vi "Test Convert.vi"(11 "Error in":errorcluster) -> (15 "Error out":errorcluster)   [LabVIEW 2020, in "CelsiusToFarenheitTests.lvlib"]
doc: "This VI is to validate Celsius to farenheit"
uses:
  CelsiusToFarenheitTests.lvlib
  <vilib>/SLL Drona/APIs/Stimulus/ControlValue/ValueSignalByPathString.vi
  <vilib>/SLL Drona/APIs/Assert/AssertControlValue/AlmostEqual.vi
  <vilib>/SLL Drona/APIs/Stimulus/VI/CloseVI.vi
  <vilib>/SLL Drona/Drona.lvlib
  <vilib>/addons/_JKI Toolkits/Caraya/classes/Test/Test.lvclass
  <vilib>/SLL Drona/APIs/Stimulus/ControlValue/ControlValue.lvlib
  <vilib>/SLL Drona/APIs/Assert/AssertControlValue/AssertControlValue.lvlib
  <vilib>/SLL Drona/APIs/Stimulus/VI/VI.lvlib
panel:
  # "CELSIUS TO FARENHEIT TEST"
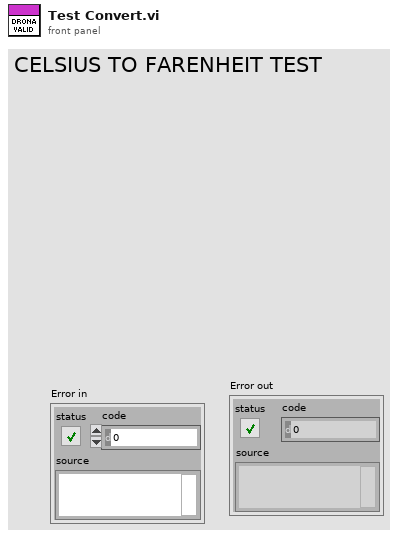
[diagram p1: front panel]
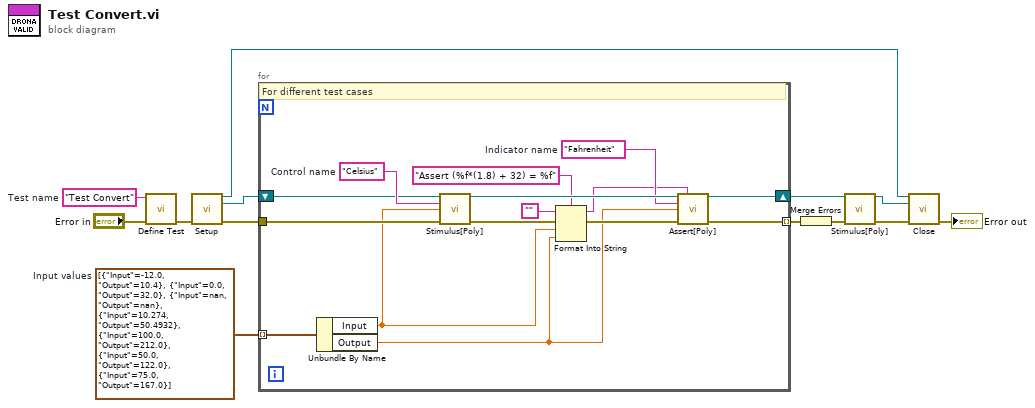
[diagram p0: block diagram]
diagram:
  w10 = "Test Convert"  # Test name
  w9 = cluster{"Input":dbl, "Output":dbl}[] [{"Input"=-12.0, "Output"=10.4}, {"Input"=0.0, "Output"=32.0}, {"Input"=nan, "Output"=nan}, {"Input"=10.274, "Output"=50.4932}, {"Input"=100.0, "Output"=212.0}, {"Input"=50.0, "Output"=122.0}, {"Input"=75.0, "Output"=167.0}]  # Input values
  n1 = call <vilib>:"Define Test.vi"("error in (no error)"="Error in", "Label (VI Title)"=w10) -> ("error out"=w12:errorcluster)  [unwired: 9 in]
  n2 = call <vilib>:"Setup.vi"("error in"=w12) -> ("Application Ref"=w7:refnum<vi>, "VI Reference Out"=w8:refnum<vi>, "error out"=w11:errorcluster)  [unwired: 12 in]
  n3 = for {
    tunnel: w9 -> [w27] mode=indexing
    shift-right: [w17] -> w6
    shift-left: w8 -> [w25]
    tunnel: w11 -> [w28]
    tunnel: [w15] -> w2 mode=indexing
    w18 = "Fahrenheit"  # Indicator name
    w26 = "Celsius"  # Control name
    # "For different test cases"
    n4 = Unbundle By Name(w27) -> ("Input"=w14:dbl, "Output"=w19:dbl)
    n5 = call-poly <vilib>:"Stimulus[Poly].vi"("VI Reference In"=w25, "Control Path"=w26, "Value (Signaling)"=w14, "error in"=w28) -> ("VI Reference Out"=w21:refnum<vi>, "error out"=w23:errorcluster)  [unwired: 10 in]
    n6 = Format Into String(format string="Assert (%f*(1.8) + 32) = %f", initial string="", error in=w23, w14, w19) -> (resulting string=w16:string, error out=w22:errorcluster)
    n7 = call-poly <vilib>:"Assert[Poly].vi"("VI Reference In"=w21, "Test Label"=w16, "Control Path"=w18, "Control Value"=w19, "Error In"=w22) -> ("VI Reference Out"=w17:refnum<vi>, "Error Out"=w15:errorcluster)  [unwired: 9 in]
  }
  n8 = Merge Errors(w2) -> (w1:errorcluster)
  n9 = call-poly <vilib>:"Stimulus[Poly].vi"("VI Reference In"=w6, "error in"=w1) -> ("VI Reference Out"=w5:refnum<vi>, "error out"=w4:errorcluster)  [unwired: 12 in]
  n10 = call <vilib>:"Close.vi"("Application Ref"=w7, "VI Reference"=w5, "error in"=w4) -> ("error out"=→"Error out":errorcluster)  [unwired: 12 in]
